vi "Graph_Create.vi"(0 "reference":refnum<class "Graph.lvclass">, 5 "error in (no error)":errorcluster, 6 "GoopReferenceIn":T1) -> (14 "reference out":refnum<class "Graph.lvclass">, 16 "# of objects":i32, 19 "error out":errorcluster)   [LabVIEW 2012, in "Graph.lvclass"]
doc: "Creates and initializes a new Graph object.\n\nThis object should be destroyed using a Graph destructor VI.\n\n[GOOP 2.1]"
uses:
  <resource>/Framework/Providers/Open_GDS/UML/Graph_class/Graph.lvclass
  <resource>/Framework/Providers/Open_GDS/UML/Graph_class/ObjectReference.ctl
  <resource>/Framework/Providers/Open_GDS/UML/AbstractNode_class/AbstractNode.lvclass
  <resource>/Framework/Providers/Open_GDS/UML/AbstractEdge_class/AbstractEdge.lvclass
panel:
  # "The input reference should only\nbe wired when this method is called\nby a sub class constructor."
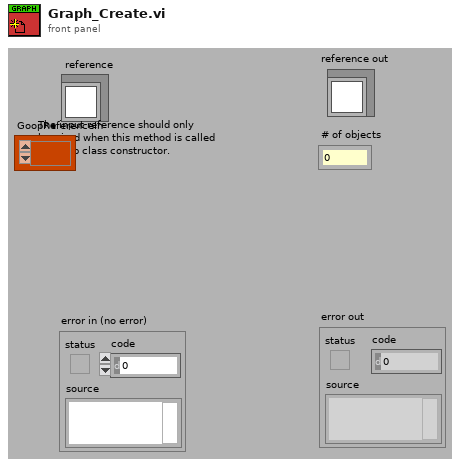
[diagram p1: front panel]
types:
  T1 = typedef "Graph.lvclass/ObjectReference.ctl" = refnum<k1>
  T2 = typedef "Graph.lvclass/ObjectAttributes.ctl" = cluster{"nodes":refnum<class "AbstractNode.lvclass">[], "edges":refnum<class "AbstractEdge.lvclass">[], "nodesToBeRemoved":refnum<class "AbstractNode.lvclass">[], "edgesToBeRemoved":refnum<class "AbstractEdge.lvclass">[], "needsLayout":bool, "LayoutNodes":refnum<class "AbstractNode.lvclass">[]}
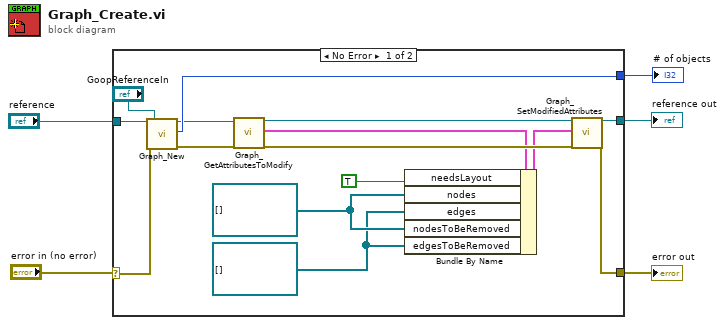
[diagram p0: block diagram]
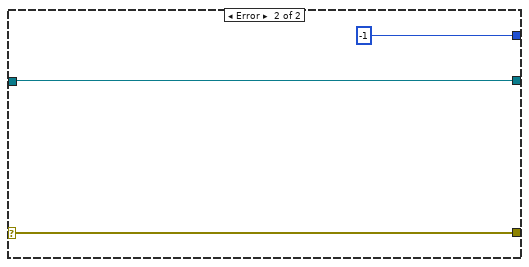
[diagram p2: hidden frame]
diagram:
  n1 = case shown="No Error" "error in (no error)" {
    selector: "error in (no error)" -> [w20 w22]
    tunnel: [w13 w21] -> w5
    tunnel: [w18 w22] -> w4
    tunnel: [w19 -1 ("Nr of open handles")] -> w3
    tunnel: "reference" -> [w12 w21]
    frame No Error {
      w6 = refnum<class "AbstractEdge.lvclass">[] [] ("edges")
      w7 = refnum<class "AbstractNode.lvclass">[] [] ("nodes")
      n2 = call <resource>:"Graph_New.vi"("reference in"=w12, "error in (no error)"=w20, "GoopReferenceIn"="GoopReferenceIn") -> ("reference out"=w15:refnum<class "Graph.lvclass">, "# of objects"=w19:i32, "error out"=w17:errorcluster)  [unwired: 2 in, 12 out]
      n3 = call <resource>:"Graph_GetAttributesToModify.vi"("reference in"=w15, "error in (no error)"=w17) -> ("reference out"=w14:refnum<class "Graph.lvclass">, "Attributes"=w11:T2, "error out"=w16:errorcluster)  [unwired: 1 in, 14 out]
      n4 = Bundle By Name(cluster=w11, "needsLayout"=TRUE, "nodes"=w7, "edges"=w6, "nodesToBeRemoved"=w7, "edgesToBeRemoved"=w6) -> (w10:T2)
      n5 = call <resource>:"Graph_SetModifiedAttributes.vi"("reference in"=w14, "Attributes"=w10, "error in (no error)"=w16) -> ("reference out"=w13:refnum<class "Graph.lvclass">, "error out"=w18:errorcluster)  [unwired: 3 in, 12 out]
    }
    frame Error {
    }
  }
  "error out" <- w4
  "reference out" <- w5
  "# of objects" <- w3
